vi "Manipulation2.vi"() -> ()   [LabVIEW 2017]
panel:
  in  "stop":bool
  in  "Tab Control":enum32{"Page 1", "Page 2"}(tab)
  out "Déroule Graph":dbl[](graph)
  out "XY Graph":cluster{dbl[], dbl[]}(graph)
  out "y":dbl[](array[numeric])
  out "x":dbl[](array[numeric])
  in  "Nombre de points":dbl
  in  "Fréquence":dbl
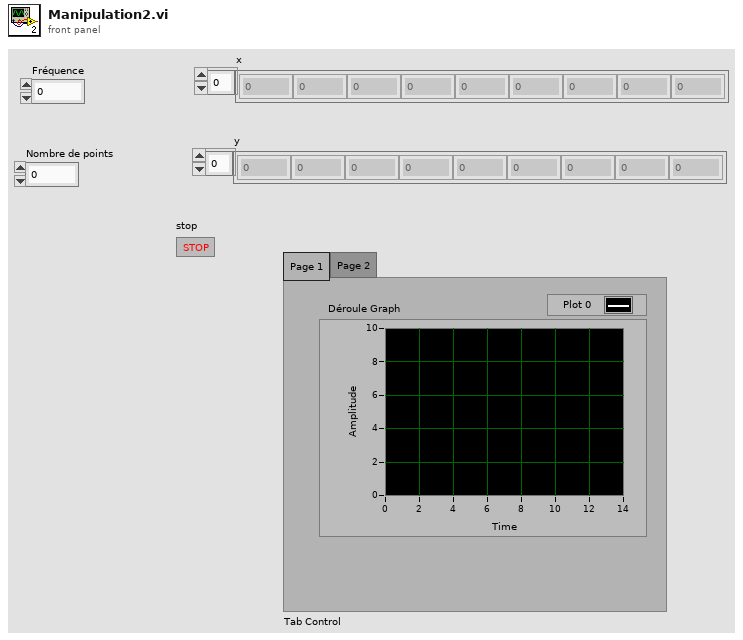
[diagram p1: front panel]
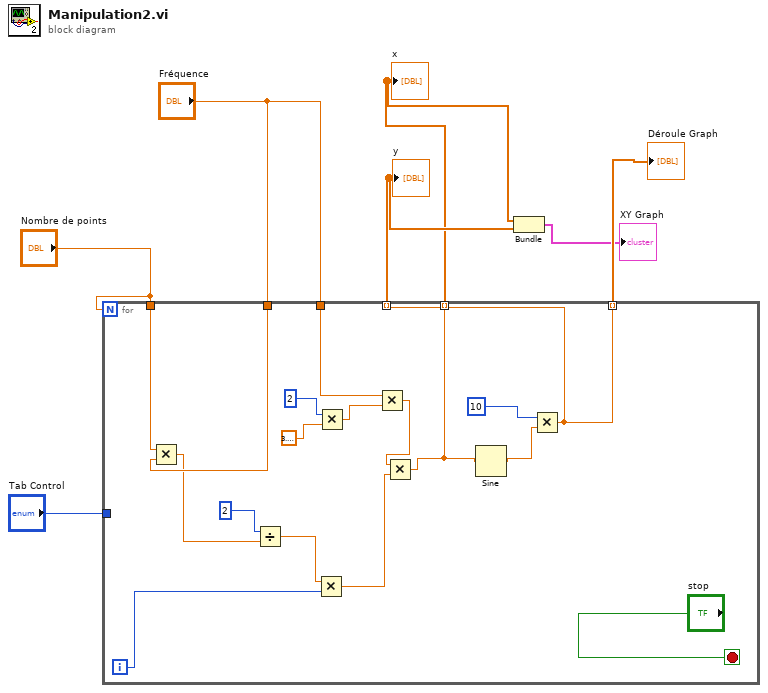
[diagram p0: block diagram]
diagram:
  n1 = for {
    N: "Nombre de points" -> [_]
    tunnel: "Fréquence" -> [w11]
    tunnel: [w18] -> w5 mode=indexing
    tunnel: [w18] -> w7 mode=indexing
    tunnel: [w14] -> w4 mode=indexing
    tunnel: "Nombre de points" -> [w12]
    tunnel: "Fréquence" -> [w8]
    tunnel: "Tab Control" -> [_]
    i -> [w19]
    stop <- "stop" stop-if-true
    n2 = Multiply(x=w12, y=w11) -> (x*y=w10:dbl)
    n3 = Divide(x=2, y=w10) -> (x/y=w9:dbl)
    n4 = Multiply(x=w9, y=w19) -> (x*y=w17:dbl)
    n5 = Multiply(x=2, y=3.141592653589793) -> (x*y=w21:dbl)
    n6 = Multiply(x=w8, y=w21) -> (x*y=w16:dbl)
    n7 = Multiply(x=w16, y=w17) -> (x*y=w14:dbl)
    n8 = Sine(x=w14) -> (sin(x)=w15:dbl)
    n9 = Multiply(x=10, y=w15) -> (x*y=w18:dbl)
  }
  "x" <- w4
  "y" <- w5
  "Déroule Graph" <- w7
  n10 = Bundle(w4, w5) -> (→"XY Graph":cluster{dbl[], dbl[]})  [unwired: 1 in]
